vi "CANcoderSet.vi"   [LabVIEW 2023]
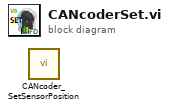
[diagram p0: block diagram]
diagram:
  n1 = call <vilib>:"CANcoder_SetSensorPosition.vi"() -> ()  [unwired: 11 in, 1 out]
